vi "LvMPDC_SUB_SendCmdAndRecvReply.vi"(6 "timeout_ms":i32=3000, 8 "error in (no error)":errorcluster, 9 "ReadBytes":i32=10240, 10 "Command":string="ping", 11 "Connect ID":refnum<k5>) -> (0 "error out":errorcluster, 2 "Reply":string, 3 "Connect ID out":refnum<k5>)   [LabVIEW 2012]
uses:
  <vilib>/Utility/error.llb/whitespace.ctl
panel:
  out "Recv String":string
  # "LvMPDC:: Send Command and ReceiveReply"
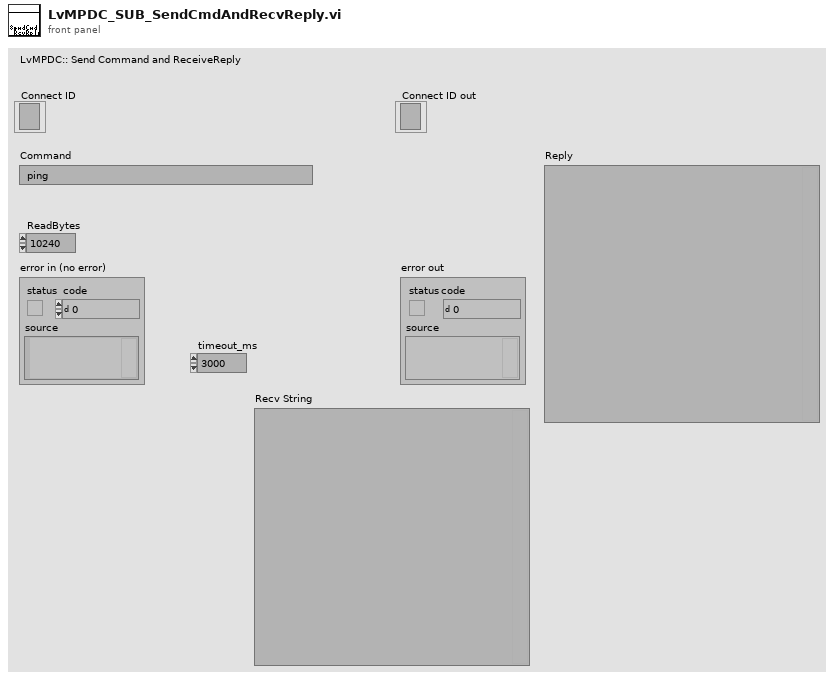
[diagram p1: front panel]
types:
  T1 = enum16{"Standard", "Buffered", "CRLF", "Immediate"}
  T2 = typedef "whitespace.ctl" = u16
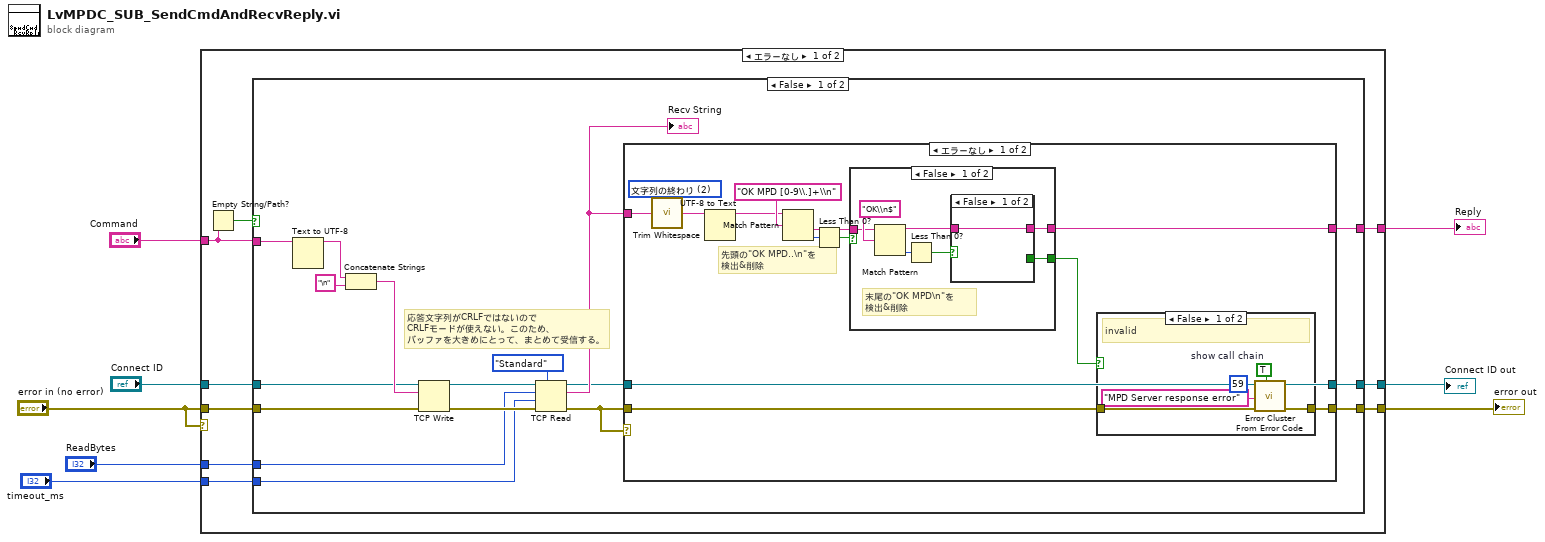
[diagram p0: block diagram]
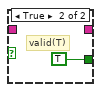
[diagram p3: hidden frame]
diagram:
  n1 = case shown="エラーなし" "error in (no error)" {
    tunnel: "Connect ID" -> [w17 w68]
    tunnel: "error in (no error)" -> [w16 w67]
    tunnel: [w15 w68] -> w7
    tunnel: [w9 w67] -> w6
    tunnel: [w10 _] -> w4
    tunnel: "Command" -> [w14 _]
    tunnel: "timeout_ms" -> [w12 _]
    tunnel: "ReadBytes" -> [w11 _]
    frame No Error {
      n2 = Empty String/Path?(string/path=w14) -> (empty?=w13:bool)
      n3 = case shown="FALSE" w13 {
        tunnel: w17 -> [w29 w66]
        tunnel: w16 -> [w28 w65]
        tunnel: [w19 w66] -> w15
        tunnel: w14 -> [w26 _]
        tunnel: w12 -> [w25 _]
        tunnel: w11 -> [w24 _]
        tunnel: [w22 _] -> w10
        tunnel: [w18 w65] -> w9
        frame False {
          # "応答文字列がCRLFではないので\nCRLFモードが使えない。このため、\nバッファを大きめにとって、まとめて受信する。"
          n4 = Text to UTF-8(11:w26) -> (3:w30:string)  [unwired: 1 in, 1 out]
          n5 = Concatenate Strings(w30, "\n" ("データ入力")) -> (w31:string)
          n6 = TCP Write(connection ID=w29, data in=w31, error in (no error)=w28) -> (connection ID out=w34:refnum<k5>, error out=w27:errorcluster)  [unwired: 1 in, 1 out]
          n7 = TCP Read(connection ID=w34, bytes to read=w24, error in (no error)=w27, 7:T1."Standard" ("モード（標準）"), 9:w25) -> (connection ID out=w21:refnum<k5>, data out=w23:string, error out=w20:errorcluster)
          "Recv String" <- w23
          n8 = case shown="エラーなし" w20 {
            tunnel: w23 -> [w47 _]
            tunnel: [w39 _] -> w22
            tunnel: w21 -> [w38 w64]
            tunnel: w20 -> [w36 w63]
            tunnel: [w38 w64] -> w19
            tunnel: [w35 w63] -> w18
            frame No Error {
              w46 = T2 2 items=["両方", "文字列の先頭", "文字列の終わり"] ("location (both)")
              # "先頭の\"OK MPD..\\n\"を\n検出&削除"
              n9 = call <vilib>:"Trim Whitespace.vi"("string"=w47, "location (both)"=w46) -> ("trimmed string"=w45:string)
              n10 = UTF-8 to Text(11:w45) -> (3:w42:string)  [unwired: 1 in, 1 out]
              n11 = Match Pattern(string=w42, regular expression="OK MPD [0-9\\.]+\\n" ("正規表現")) -> (after substring=w43:string, offset past match=w41:i32)  [unwired: 1 in, 2 out]
              n12 = Less Than 0?(x=w41) -> (x < 0?=w40:bool)
              n13 = case shown="FALSE" w40 {
                tunnel: w43 -> [w59 _]
                tunnel: [w55 _] -> w39
                tunnel: [w54 _] -> w37
                frame False {
                  # "末尾の\"OK MPD\\n\"を\n検出&削除"
                  n14 = Match Pattern(string=w59, regular expression="OK\\n$" ("正規表現")) -> (before substring=w56:string, offset past match=w58:i32)  [unwired: 1 in, 2 out]
                  n15 = Less Than 0?(x=w58) -> (x < 0?=w57:bool)
                  n16 = case shown="FALSE" w57 {
                    tunnel: w56 -> [w61 _]
                    tunnel: [w61 _] -> w55
                    tunnel: [_ TRUE] -> w54
                    frame False {
                    }
                    frame True {
                      # "valid(T)"
                    }
                  }
                }
                frame True {
                }
              }
              n17 = case shown="FALSE" w37 {
                tunnel: w36 -> [w51 w53]
                tunnel: [w50 w53] -> w35
                frame False {
                  w52 = TRUE  # show call chain
                  # "invalid"
                  n18 = call <vilib>:"Error Cluster From Error Code.vi"("show call chain? (False)"=w52, "error in (no error)"=w51, "error message (\"\")"="MPD Server response error", "error code (0)"=59) -> ("error out"=w50:errorcluster)  [unwired: 5 in]
                }
                frame True {
                  # "valid"
                }
              }
            }
            frame Error {
            }
          }
        }
        frame True {
        }
      }
    }
    frame Error {
    }
  }
  "Connect ID out" <- w7
  "error out" <- w6
  "Reply" <- w4
